vi "Dictionary Get Instance Semaphore RefNum__ogtk.vi"(8 "error out":errorcluster, 11 "Object RefNum":T1) -> (0 "error in (no error)":errorcluster, 2 "semaphore":T2, 3 "dup Object RefNum":T1)   [LabVIEW 2017]
uses:
  <userlib>/_OpenG.lib/dictionary/dictionary.llb/Dictionary Object RefNum__ogtk.ctl
  <userlib>/_OpenG.lib/dictionary/dictionary.llb/Dictionary Object RefNum - Enum__ogtk.ctl
panel:
  # "<VI Name>\n\n<VI Description>\n\nPlease visit http://www.OpenG.org to learn about the\nOpen Source LabVIEW software movement.\n\nNOTICE -- YOU MUST LEAVE THIS NOTICE IN PLACE.  PER THE TERMS OF THE LICENSE BELOW, YOU MAY SUBLICENSE THIS SOFTWARE \nIN ANY WAY THAT DOES NOT CONFLICT WITH THIS LICENSE.\n\n### BSD License (http://www.opensource.org/licenses/bsd-license.php) Begin ###\n \nCopyright (c) 2003, Jim Kring <jim@jimkring.com>\n\nAll rights reserved.\n\nRedistribution and use in source and binary forms, with or without modification, are permitted provided that the following conditions are met:\n\n    * Redistributions of source code must retain the above copyright notice, this list of conditions and the following disclaimer.\n    * Redistributions in binary form must reproduce the above copyright notice, this list of conditions and the following disclaimer in the \n       documentation and/or other materials provided with the distribution.\n    * Neither the name of SciWare, James Kring, Inc., nor the names of its contributors may be used to endorse or promote products derived \n       from this software without specific prior written permission.\n\nTHIS SOFTWARE IS PROVIDED BY THE COPYRIGHT HOLDERS AND CONTRIBUTORS \"AS IS\" AND ANY EXPRESS OR IMPLIED WARRANTIES, \nINCLUDING, BUT NOT LIMITED TO, THE IMPLIED WARRANTIES OF MERCHANTABILITY AND FITNESS FOR A PARTICULAR PURPOSE ARE \nDISCLAIMED. IN NO EVENT SHALL THE COPYRIGHT OWNER OR CONTRIBUTORS BE LIABLE FOR ANY DIRECT, INDIRECT, INCIDENTAL,\n SPECIAL, EXEMPLARY, OR CONSEQUENTIAL DAMAGES (INCLUDING, BUT NOT LIMITED TO, PROCUREMENT OF SUBSTITUTE GOODS OR \nSERVICES; LOSS OF USE, DATA, OR PROFITS; OR BUSINESS INTERRUPTION) HOWEVER CAUSED AND ON ANY THEORY OF LIABILITY, \nWHETHER IN CONTRACT, STRICT LIABILITY, OR TORT (INCLUDING NEGLIGENCE OR OTHERWISE) ARISING IN ANY WAY OUT OF THE USE \nOF THIS SOFTWARE, EVEN IF ADVISED OF THE POSSIBILITY OF SUCH DAMAGE.\n\n### BSD License End ###"
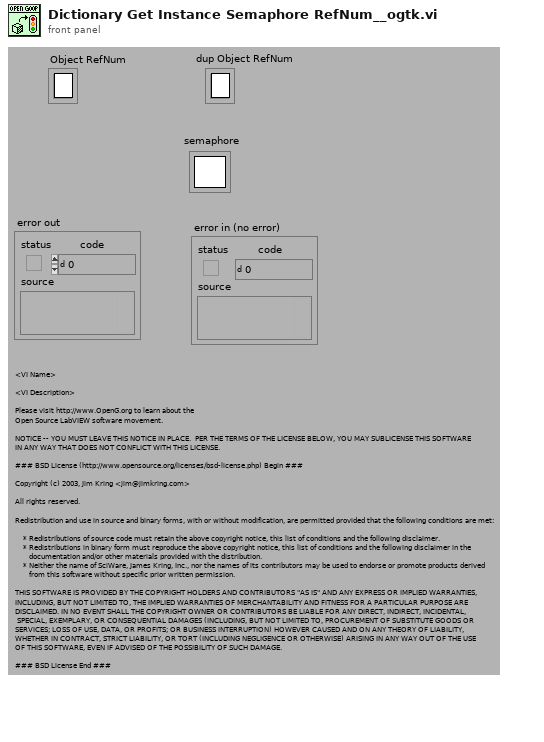
[diagram p1: front panel]
types:
  T1 = typedef "Dictionary Object RefNum__ogtk.ctl" = refnum<k1>
  T2 = typedef "Semaphore RefNum" = refnum<k1>
  T3 = typedef "Dictionary Object RefNum - Enum__ogtk.ctl" = enum16{"Dictionary"}
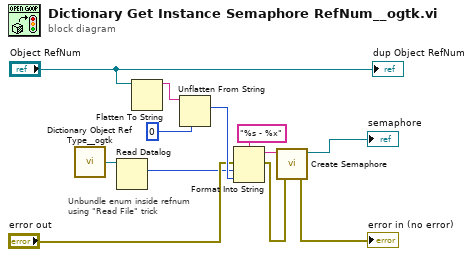
[diagram p0: block diagram]
diagram:
  # "Unbundle enum inside refnum using \"Read File\" trick"
  n1 = call <userlib>:"Dictionary Object Ref Type__ogtk.vi"() -> ("Object RefNum Type"=w2:T1)  [unwired: 5 in]
  n2 = Read Datalog(7:w2) -> (2:w1:T3)  [unwired: 2 in, 2 out]
  n3 = Flatten To String(anything="Object RefNum") -> (data string=w12:string)  [unwired: 3 in, 2 out]
  n4 = Unflatten From String(type=u32 0 ("input 2"), binary string=w12) -> (value=w11:u32)  [unwired: 3 in, 2 out]
  n5 = Format Into String(format string="%s - %x", error in="error out", w1, w11) -> (resulting string=w8:string, error out=w9:errorcluster)  [unwired: 1 in]
  n6 = call <vilib>:"Create Semaphore.vi"("error in (no error)"=w9, "name (unnamed)"=w8) -> ("error out"=→"error in (no error)":errorcluster, "semaphore"=→"semaphore":T2)  [unwired: 3 in, 1 out]
  "dup Object RefNum" <- "Object RefNum"
